vi "Drive Angle.vi"(4 "Timeout ms (-1)":i32=-1, 6 "Wait for Completion? (F)":bool, 7 "Force? (F)":bool, 8 "error in":errorcluster, 9 "Gyro ms ago":u32, 10 "Drive Magnitude":dbl, 11 "Angle":dbl) -> (0 "error out":errorcluster)   [LabVIEW 2016, in "Drive System.lvlib"]
uses:
  Drive System.lvlib
  Private/Varient Cmd Types/Drive Angle Magnitude.ctl
  Private/DriveCmd.ctl
  Private/DriveCmdList.ctl
  Private/Drive Refs/Drive Angle Magnitude.vi
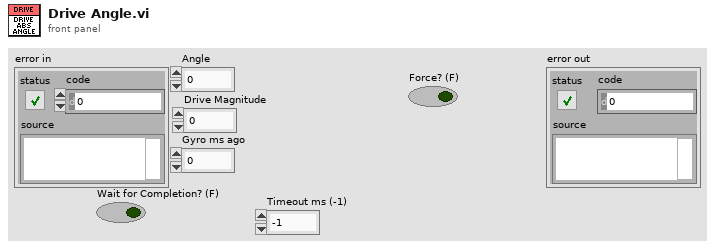
[diagram p1: front panel]
types:
  T1 = typedef "Drive System.lvlib/Drive Angle Magnitude.ctl" = cluster{"Angle":dbl, "Drive Magnitude":dbl, "Get ms ago":u32}
  T2 = typedef "Drive System.lvlib/DriveCmd.ctl" = cluster{"cmd":T3, "data":variant, "Force? (F)":bool, "Lock":string}
  T3 = typedef "Drive System.lvlib/DriveCmdList.ctl" = enum16{"Idle", "Cleanup", "Drive For Time", "Follow Path Speed Control", "Follow Path", "Drive Tank", "Drive Angle Mag", "Drive Arcade", "Drive Ref", "Unlock", "Lock"}
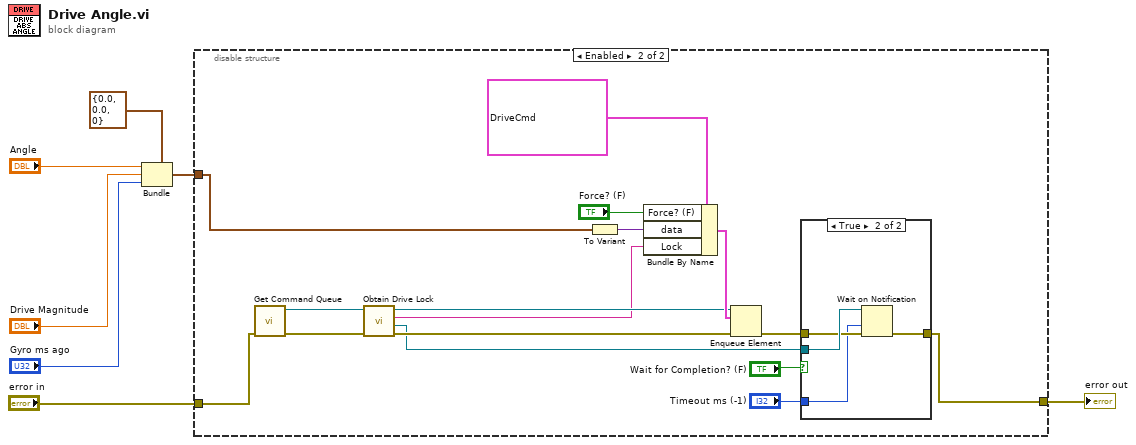
[diagram p0: block diagram]
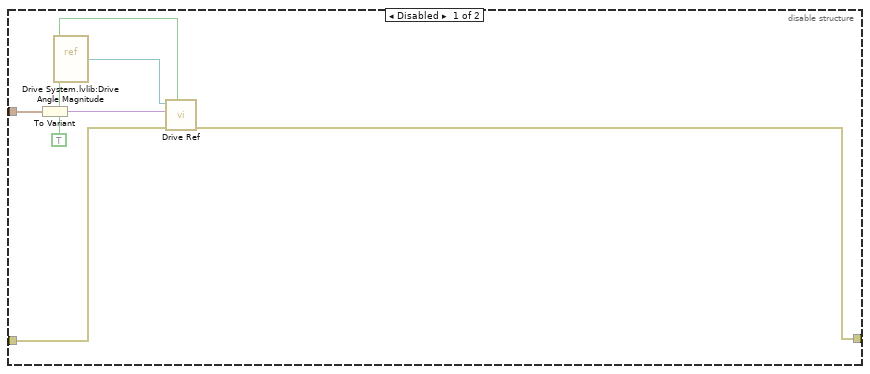
[diagram p2: hidden frame]
diagram:
  n1 = Bundle(cluster=T1 {"Angle"=0.0, "Drive Magnitude"=0.0, "Get ms ago"=0} ("Cluster"), "Angle"="Angle", "Drive Magnitude"="Drive Magnitude", "Get ms ago"="Gyro ms ago") -> (w5:T1)
  n2 = disable-structure shown="Enabled" {
    disable-tunnel: [w12 w16] -> w7
    disable-tunnel: "error in" -> [w11 w15]
    disable-tunnel: w5 -> [w9 w14]
    frame Disabled {
      n3 = To Variant(anything=w9) -> (Variant=w13:variant)
      n4 = vi-ref "Drive System.lvlib:Drive Angle Magnitude.vi"() -> (w8:refnum<vi>)
      n5 = call "Drive Ref.vi"("Locking? (F)"=TRUE, "error in"=w11, "Data"=w13, "VI Refnum"=w8) -> ("error out"=w12:errorcluster)  [unwired: 6 in, 1 out]
    }
    frame Enabled {
      n6 = call "Get Command Queue.vi"("error in (no error)"=w15) -> ("error out"=w29:errorcluster, "Queue out"=w28:refnum<queue>)  [unwired: 9 in]
      n7 = call "Obtain Drive Lock.vi"("error in"=w29, "Queue in"=w28) -> ("error out"=w23:errorcluster, "notifier out"=w19:refnum<notifier>, "Lock"=w21:string, "queue out"=w22:refnum<queue>)  [unwired: 6 in]
      n8 = To Variant(anything=w14) -> (Variant=w26:variant)
      n9 = Bundle By Name(cluster=T2 {"cmd"=enum."Drive Angle Mag", "data"=variant, "Force? (F)"=FALSE, "Lock"=""} ("element"), "Force? (F)"="Force? (F)", "data"=w26, "Lock"=w21) -> (w27:T2)
      n10 = Enqueue Element(queue=w22, element=w27, error in (no error)=w23) -> (error out=w20:errorcluster)  [unwired: 1 in, 2 out]
      n11 = case shown="True" "Wait for Completion? (F)" {
        tunnel: w20 -> [w30 w33]
        tunnel: w19 -> [_ w34]
        tunnel: [w30 w32] -> w16
        tunnel: "Timeout ms (-1)" -> [_ w31]
        frame False {
        }
        frame True {
          n12 = Wait on Notification(notifier=w34, timeout in ms (-1)=w31, error in (no error)=w33) -> (error out=w32:errorcluster)  [unwired: 1 in, 3 out]
        }
      }
    }
  }
  "error out" <- w7
